vi "RSZVB Set Simultaneous Measurement Frequency Offset State.vi"(8 "error in (no error)":errorcluster {"code" format="%.0x"}, 9 "State (Off)":bool, 10 "Channel (1)":i32=1, 11 "VISA resource name":refnum<visa-resource-name>) -> (0 "error out":errorcluster {"code" format="%.0x"}, 3 "VISA resource name out":refnum<visa-resource-name>)   [LabVIEW 2011]
doc: "This VI activates/deactivates the Simultaneous Measurement with Frequency Offset which performs measurements within different port groups in parallel while applying different frequency offsets to the measurements in different port groups.\n\nRemote-control command(s):\nSOURce<Ch>:GROup:SIMultaneous:FOFFset[:STATe]"
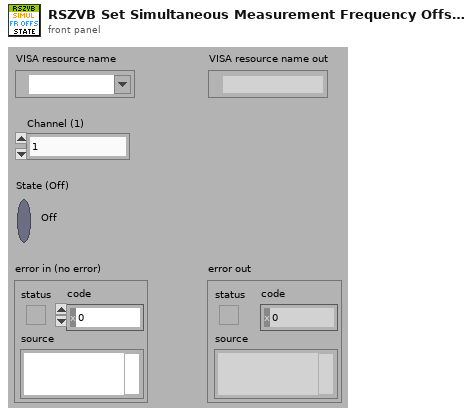
[diagram p1: front panel]
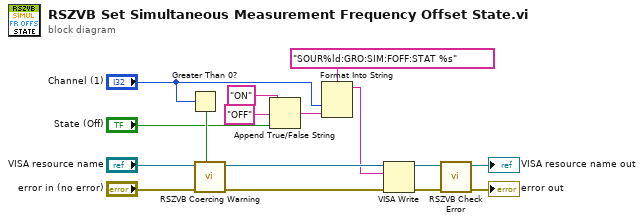
[diagram p0: block diagram]
diagram:
  n1 = Greater Than 0?(x="Channel (1)") -> (x > 0?=w10:bool)
  n2 = call "RSZVB Coercing Warning.vi"("In Range?"=w10, "error in (no error)"="error in (no error)", "VISA session"="VISA resource name") -> ("error out"=w14:errorcluster, "dup VISA session"=w15:refnum<visa-resource-name>)  [unwired: 7 in]
  n3 = Append True/False String(1:"State (Off)", 2:"OFF", 3:"ON") -> (0:w7:string)  [unwired: 1 in]
  n4 = Format Into String(format string="SOUR%ld:GRO:SIM:FOFF:STAT %s", "Channel (1)", w7) -> (resulting string=w11:string)  [unwired: 2 in, 1 out]
  n5 = VISA Write(VISA resource name=w15, write buffer=w11, error in (no error)=w14) -> (VISA resource name out=w12:refnum<visa-resource-name>, error out=w13:errorcluster)  [unwired: 1 out]
  n6 = call "RSZVB Check Error.vi"("error in (no error)"=w13, "VISA session"=w12) -> ("error out"=→"error out":errorcluster, "dup VISA session"=→"VISA resource name out":refnum<visa-resource-name>)  [unwired: 8 in]
